vi "Gain_Schedule.vi"(11 "Initialize?":bool) -> (1 "Outpower?":bool, 2 "Resistance?":bool, 3 "Array 2":T1(array[cluster]))   [LabVIEW 2009]
panel:
  in  "I or P":bool
  in  "T or R":bool
  in  "Done":bool
  in  "Array":T2(array[cluster])
  # "Choose a PID Gain Schedule:\n  -  Choose PID parameters for different temperature/resistance regimes.\n  -  If the temperature or resistance exceeds the highest maximum value, the PID \n     parameters corresponding to the highest maximum value will continue to be used.\n  -  Choose whether gain is a function of thermocouple temperature or measured \n     resistance using the switch below.\n  -  Choose whether the PID algorithm calculates a current or a power that then gets \n     converted to a current."
  # "Gain as a function of:"
  # "Temperature [C]"
  # "Time [s]"
  # "PID calculates:"
  # "Current"
  # "Power => Current"
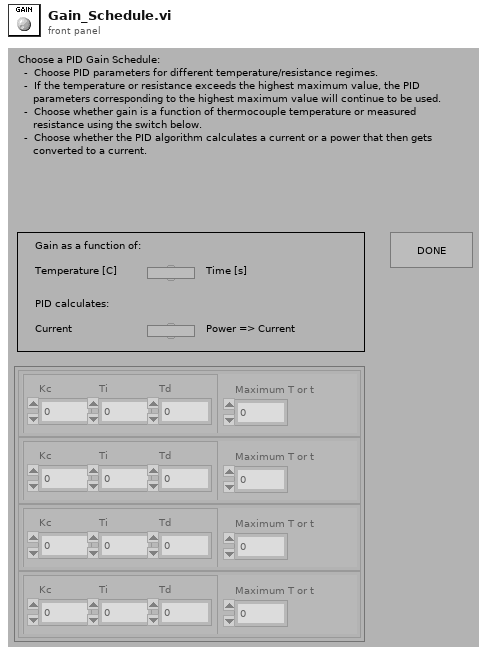
[diagram p1: front panel]
types:
  T1 = cluster{"Parameters":cluster{"Kc":dbl, "Ti":dbl, "Td":dbl}, "Maximum Temp [C]":dbl}[]
  T2 = cluster{"Parameters":cluster{"Kc":dbl, "Ti":dbl, "Td":dbl}, "Maximum T or t":dbl}[]
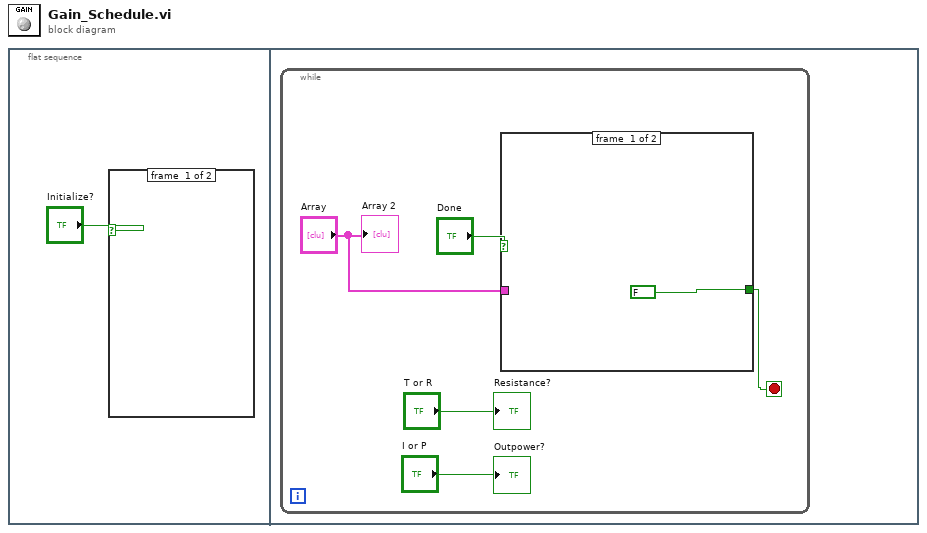
[diagram p0: block diagram]
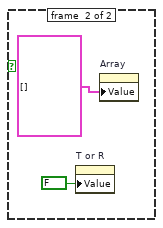
[diagram p2: hidden frame]
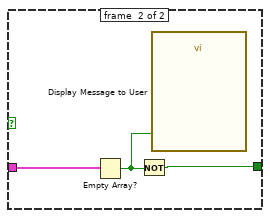
[diagram p3: hidden frame]
diagram:
  n1 = flat-sequence {
    frame #0 {
      n2 = case shown="True" "Initialize?" {
        frame #0 {
        }
        frame #1 {
          n3 = property on="T or R" class="Bool (strict)"("Value"=FALSE ("T or R")) -> ()  [unwired: 2 in, 2 out]
          n4 = property on="Array" class="Arr (strict)"("Value"=T1 [] ("Array")) -> ()  [unwired: 2 in, 2 out]
        }
      }
    }
    frame #1 {
      n5 = while {
        stop <- w6 stop-if-true
        n6 = case shown="True" "Done" {
          tunnel: "Array" -> [_ w12]
          tunnel: [FALSE w11] -> w6
          frame #0 {
          }
          frame #1 {
            n7 = Empty Array?(array=w12) -> (empty?=w10:bool)
            n8 = Not(x=w10) -> (.not. x?=w11:bool)
            n9 = call "Display Message to User"("Enable"=w10) -> ()  [unwired: 9 in, 2 out]
          }
        }
        "Array 2" <- "Array"
        "Resistance?" <- "T or R"
        "Outpower?" <- "I or P"
      }
    }
  }
